vi "ui_Library One Button Dialog.vi"(1 "button name (\"OK\")":string="OK", 2 "message":string) -> (0 "true":bool)   [LabVIEW 2012]
doc: "Drop-in replacement for LabVIEW's One Button Dialog\" which, at least up to LabVIEW version 7.1, has the nasty property that it blocks the user interface thread while open. The UI thread is required not just for display updates but also for VI loading and instantiation. Thus, using the standard One Button Dialog\" might prevent essential background tasks from doing their job. Since this subVI is implemented in LabVIEW, it does not suffer from this problem. Its connector pane layout is identical so that a simple diagram replace will work."
panel:
  out "message box":string
  in  "T button":bool
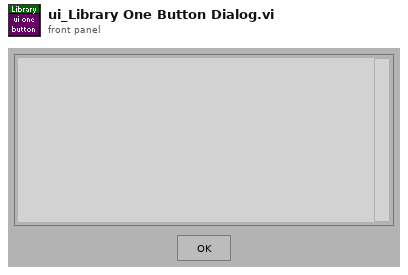
[diagram p1: front panel]
types:
  T1 = typedef "eventvkey.ctl" = enum16{"ASCII", "Enter", "Return", "Shift", "Ctrl", "Alt", "Cmd", "Opt", "Caps", "NumLock", "Clear", "Break", "Up", "Down", "Left", "Right", "Insert", "Delete", "Home", "End", "PageUp", "PageDown", "Escape", "Help", "Pause", "ScrollLock", "F1", "F2", "F3", "F4", "F5", "F6", "F7", "F8", "F9", "F10", "F11", "F12", "F13", "F14", "F15", "F16", "F17", "F18", "F19", "F20", "F21", "F22", "F23", "F24", "Play", "VolumeUp", "VolumeDown", "Mute", "Two Byte Char"}
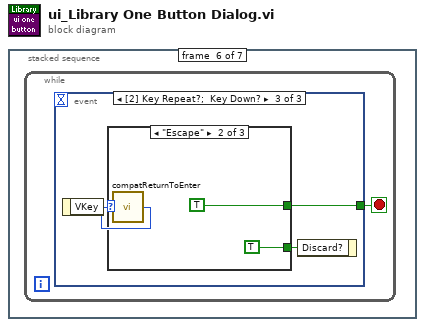
[diagram p0: block diagram]
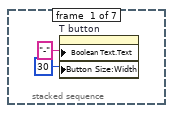
[diagram p2: hidden frame]
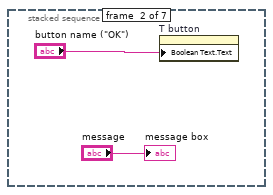
[diagram p3: hidden frame]
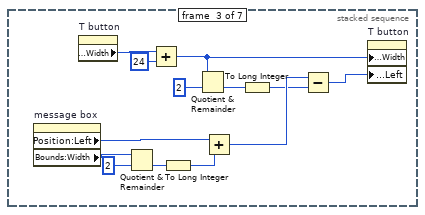
[diagram p4: hidden frame]
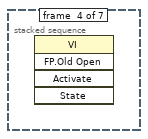
[diagram p5: hidden frame]
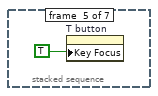
[diagram p6: hidden frame]
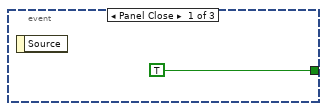
[diagram p7: hidden frame]
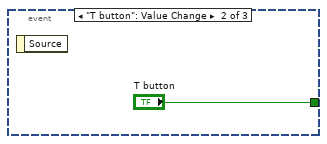
[diagram p8: hidden frame]
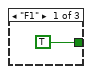
[diagram p9: hidden frame]
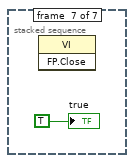
[diagram p11: hidden frame]
diagram:
  n1 = stacked-sequence {
    frame #0 {
      n2 = property on="T button" class="Bool"("Boolean Text.Text"="-", "Button Size:Width"=u32 30) -> ()  [unwired: 2 in, 2 out]
    }
    frame #1 {
      n3 = property on="T button" class="Bool"("Boolean Text.Text"="button name (\"OK\")") -> ()  [unwired: 2 in, 2 out]
      "message box" <- "message"
    }
    frame #2 {
      n4 = property on="message box" class="Str"() -> ("Position:Left"=w15:i32, "Bounds:Width"=w13:u32)  [unwired: 2 in, 2 out]
      n5 = property on="T button" class="Bool"() -> ("Button Size:Width"=w14:u32)  [unwired: 2 in, 2 out]
      n6 = Quotient & Remainder(x=w13, y=u32 2) -> (floor(x/y)=w11:u32)  [unwired: 1 out]
      n7 = Add(x=w14, y=u32 24) -> (x+y=w10:u32)
      n8 = To Long Integer(number=w11) -> (32bit integer=w16:i32)
      n9 = Quotient & Remainder(x=w10, y=u32 2) -> (floor(x/y)=w7:u32)  [unwired: 1 out]
      n10 = Add(x=w15, y=w16) -> (x+y=w8:i32)
      n11 = To Long Integer(number=w7) -> (32bit integer=w6:i32)
      n12 = Subtract(x=w8, y=w6) -> (x-y=w5:i32)
      n13 = property on="T button" class="Bool"("Button Size:Width"=w10, "Position:Left"=w5) -> ()  [unwired: 2 in, 2 out]
    }
    frame #3 {
      n14 = invoke class="VI" method="FP.Old Open"() -> ()  [unwired: 5 in, 5 out]
    }
    frame #4 {
      n15 = property on="T button" class="Bool"("Key Focus"=TRUE) -> ()  [unwired: 2 in, 2 out]
    }
    frame #5 {
      n16 = while {
        stop <- w19 stop-if-true
        n17 = event shown="[2] Key Repeat?;  Key Down?" {
          selector: _ -> [_ _ _]
          dyn-events: _ -> [_ _ _]
          timeout: _ -> [_ _ _]
          tunnel: [TRUE "T button" w23] -> w19
          event Panel Close {
            n18 = event-data() -> ()  [unwired: 1 in, 1 out]
          }
          event "T button": Value Change {
            n19 = event-data() -> ()  [unwired: 1 in, 1 out]
          }
          event event type 5.0.x8000000b; Key Down? {
            n20 = event-data() -> ("VKey"=w22:T1)  [unwired: 1 in]
            n21 = call <vilib>:"compatReturnToEnter.vi"("VKey"=w22) -> ("VKey"=w25:T1)
            n22 = case shown="\"Escape\"" w25 {
              tunnel: [TRUE ("Discard?") TRUE ("Discard?") _] -> w24
              tunnel: [_ TRUE ("T button") _] -> w23
              frame "F1" {
              }
              frame "Escape" {
              }
              frame Default {
              }
            }
            n23 = event-data("Discard?"=w24) -> ()  [unwired: 1 in, 1 out]
          }
        }
      }
    }
    frame #6 {
      n24 = invoke class="VI" method="FP.Close"() -> ()  [unwired: 3 in, 3 out]
      "true" <- TRUE ("true")
    }
  }
